vi "Calc XYZ_ij.vi"(8 "theta_j":dbl, 9 "j":i32, 10 "XYZ_i":dbl[](array[numeric]), 11 "Analytical Serial Arm Class in":refnum<class "NI_Robotics_Analytical Serial Arm Class.lvclass">) -> (1 "Xstar_ij":dbl, 2 "XYZ_ij":dbl[](array[numeric]), 3 "Analytical Serial Arm Class out":refnum<class "NI_Robotics_Analytical Serial Arm Class.lvclass">)   [LabVIEW 2017, in "NI_Robotics_Analytical Serial Arm Class.lvclass"]
uses:
  <vilib>/robotics/Kinematics/Analytical/Generic/NI_Robotics_Analytical Serial Arm Class.lvclass
  c:/Program Files (x86)/National Instruments/LabVIEW 2017/vi.lib/robotics/Kinematics/Robot/NI_Robotics_Serial Robot Arm.lvclass
  <vilib>/robotics/Kinematics/Link/NI_Robotics_Link.lvclass/NI_Robotics_Link.ctl
  <vilib>/robotics/Kinematics/Link/Get Kinematic Parameters.vi
  <vilib>/robotics/Kinematics/Analytical/Generic/Accessors/Read alpha_n0.vi
  <vilib>/robotics/Kinematics/Robot/Get Links.vi
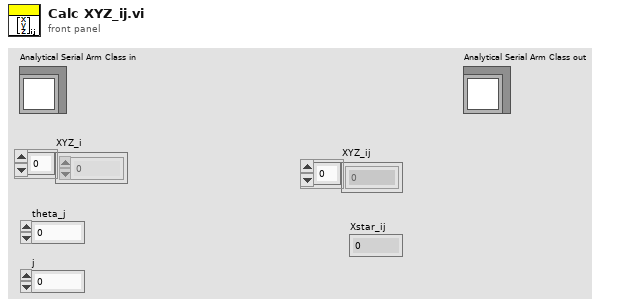
[diagram p1: front panel]
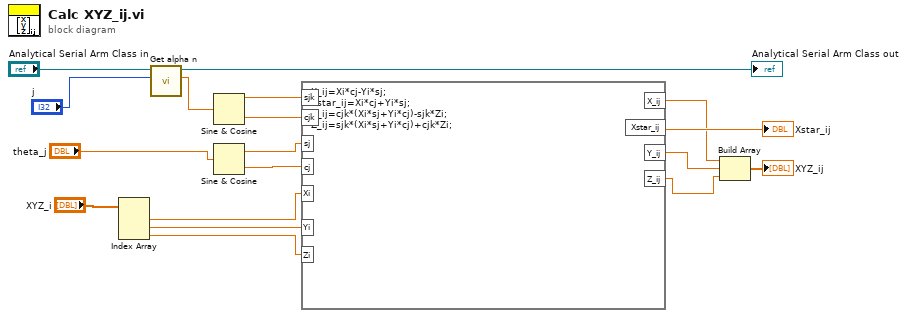
[diagram p0: block diagram]
diagram:
  n1 = Index Array(array="XYZ_i") -> (element #1=w3:dbl, element #2=w2:dbl, element #3=w1:dbl)  [unwired: 3 in]
  n2 = call <vilib>:"Get alpha n.vi"("n"="j", "Analytical Serial Arm Class in"="Analytical Serial Arm Class in") -> ("alpha n"=w15:dbl, "Analytical Serial Arm Class out"=→"Analytical Serial Arm Class out":refnum<class "NI_Robotics_Analytical Serial Arm Class.lvclass">)  [unwired: 8 in]
  n3 = Sine & Cosine(0:w15) -> (1:w12:dbl, 2:w11:dbl)
  n4 = Sine & Cosine(0:"theta_j") -> (1:w10:dbl, 2:w9:dbl)
  n5 = formula code="X_ij=Xi*cj-Yi*sj;\nXstar_ij=Xi*cj+Yi*sj;\nY_ij=cjk*(Xi*sj+Yi*cj)-sjk*Zi;\nZ_ij=sjk*(Xi*sj+Yi*cj)+cjk*Zi;"("sjk"=w12, "cjk"=w11, "sj"=w10, "cj"=w9, "Xi"=w3, "Yi"=w2, "Zi"=w1) -> ("X_ij"=w6:dbl, "Xstar_ij"=→"Xstar_ij":dbl, "Y_ij"=w7:dbl, "Z_ij"=w8:dbl)
  n6 = Build Array(w6, w7, w8) -> (→"XYZ_ij":dbl[])
